vi "Periodic Tasks.vi"(8 "error in":errorcluster) -> ()   [LabVIEW 2012]
doc: "This VI runs in parallel to other tasks. It can contain as many user-defined periodic loops as you need. These can carry out PID or other sorts of timed response."
uses:
  <vilib>/Rock Robotics/SystemInterfaces/Utilities/FPGA_UtilitiesLED Source.ctl
  <vilib>/Rock Robotics/SystemInterfaces/Utilities/FPGA_UtilitiesLED State.ctl
  <vilib>/Rock Robotics/WPI/Solenoid/WPI_SolenoidValue.ctl
  Robot Global Data.vi
  <vilib>/Rock Robotics/WPI/Solenoid/WPI_SolenoidSetEnum.vi
  <vilib>/Rock Robotics/WPI/Compressor/WPI_CompressorGetSetRefNum.vi
panel:
  out "Angle":dbl
  out "Ave Voltage":dbl
  out "Voltage":dbl
  out "PickupErrort":errorcluster
  # "AnglePot"
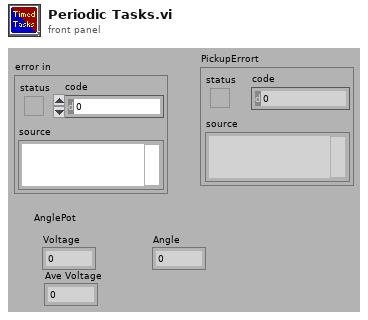
[diagram p1: front panel]
types:
  T1 = enum16{"Reset", "Ready", "Down", "Capture", "Lift", "Swing", "Release"}
  T2 = typedef "WPI_MotorControlDeviceRef.ctl" = cluster{"DeviceStatus":errorcluster, "Type":enum16{"PWM", "CAN"}, "PWM":cluster{"Digital Module":T3, "PWM Channel":T4, "DeadBand":T5}, "CAN":cluster{"Device Number":u8, "Control Mode":T6, "Semaphore":T7, "Max Vout":dbl}, "Invert":bool, "TransformRef":T8, "InvTransformRef":T8}
  T3 = typedef "FPGA_TypedefDigitalModule.ctl" = enum16{"Digital Module 1", "Digital Module 2"}
  T4 = typedef "FPGA_DIOPWMChannel.ctl" = enum8{"PWM 1", "PWM 2", "PWM 3", "PWM 4", "PWM 5", "PWM 6", "PWM 7", "PWM 8", "PWM 9", "PWM 10", "Invalid"}
  T5 = typedef "WPI_PWMDeadband.ctl" = cluster{"Name":string, "maxPositivePwm":i32, "minPositivePwm":i32, "centerPwm":i32, "maxNegativePwm":i32, "minNegativePwm":i32, "angularRange":u16}
  T6 = typedef "WPI_CANJaguar_ControlMode.ctl" = enum8{"Percent VBus", "Current", "Speed", "Position", "Voltage"}
  T7 = typedef "Semaphore RefNum" = refnum<k1>
  T8 = typedef "WPI_PWMTransform_ConPane.ctl" = refnum<vi>
  T9 = typedef "WPI_SolenoidDevRef.ctl" = cluster{"DevStatus":errorcluster, "Solenoid Module":T10, "Forward Solenoid Channel":T11, "Reverse Solenoid Channel":T11}
  T10 = typedef "FPGA_TypedefSolenoidModule.ctl" = enum16{"Solenoid Module 1", "Solenoid Module 2"}
  T11 = typedef "WPI_SolenoidChannel.ctl" = enum8{"Solenoid 1", "Solenoid 2", "Solenoid 3", "Solenoid 4", "Solenoid 5", "Solenoid 6", "Solenoid 7", "Solenoid 8", "Invalid"}
  T12 = typedef "WPI_AnalogChannelDevRef.ctl" = cluster{"DevStatus":errorcluster, "Analog Module":T13, "Analog Channel":T14}
  T13 = typedef "FPGA_TypedefAnalogModule.ctl" = enum16{"Analog Module 1", "Analog Module 2"}
  T14 = typedef "FPGA_AIChannel.ctl" = enum8{"AI 1", "AI 2", "AI 3", "AI 4", "AI 5", "AI 6", "AI 7", "AI 8", "Invalid"}
  T15 = typedef "FPGA_UtilitiesLED State.ctl" = enum16{"Off", "On", "Toggle"}
  T16 = typedef "FPGA_UtilitiesLED Source.ctl" = enum16{"User LED", "FPGA LED"}
  T17 = typedef "WPI_SolenoidValue.ctl" = enum16{"Off", "On", "Forward", "Reverse"}
  T18 = cluster{"Shoot":bool, "Enable_Targeting":bool, "Shooter":dbl, "LeadScrew":dbl, "Feed":bool, "SuctionCup":bool, "SuctionRotate":bool, "SuctionExtend":bool, "Pickup":bool, "PizzaBottom":bool, "PizzaMid":bool, "Pizza_top":bool}
  T19 = cluster{"Prox1":bool, "Prox2":bool, "Prox3":bool, "Frisbee_Catch":bool, "Frisbee_Side_Check":bool, "Shooter_Ready":bool, "LeadScrewEnd":bool}
  T20 = cluster{"PizzaLow":dbl, "PizzaMid":dbl, "PizzaTop":dbl}
  T21 = typedef "WPI_CompressorDevRef.ctl" = cluster{"DevStatus":errorcluster, "DigitalInputDevRef":T22, "RelayDevRef":T24}
  T22 = typedef "WPI_DigitalInputDevRef.ctl" = cluster{"DevStatus":errorcluster, "DIO Channel":T23, "Digital Module":T3}
  T23 = typedef "FPGA_DIOChannel.ctl" = enum8{"DIO 1", "DIO 2", "DIO 3", "DIO 4", "DIO 5", "DIO 6", "DIO 7", "DIO 8", "DIO 9", "DIO 10", "DIO 11", "DIO 12", "DIO 13", "DIO 14", "Invalid"}
  T24 = typedef "WPI_RelayDevRef.ctl" = cluster{"DevStatus":errorcluster, "Relay Channel":T25, "Digital Module":T3, "Relay Direction":T26}
  T25 = typedef "FPGA_DIORelayChannel.ctl" = enum8{"Relay 1", "Relay 2", "Relay 3", "Relay 4", "Relay 5", "Relay 6", "Relay 7", "Relay 8", "Invalid"}
  T26 = typedef "WPI_RelayDirection.ctl" = enum16{"Both directions", "Forward only", "Reverse only"}
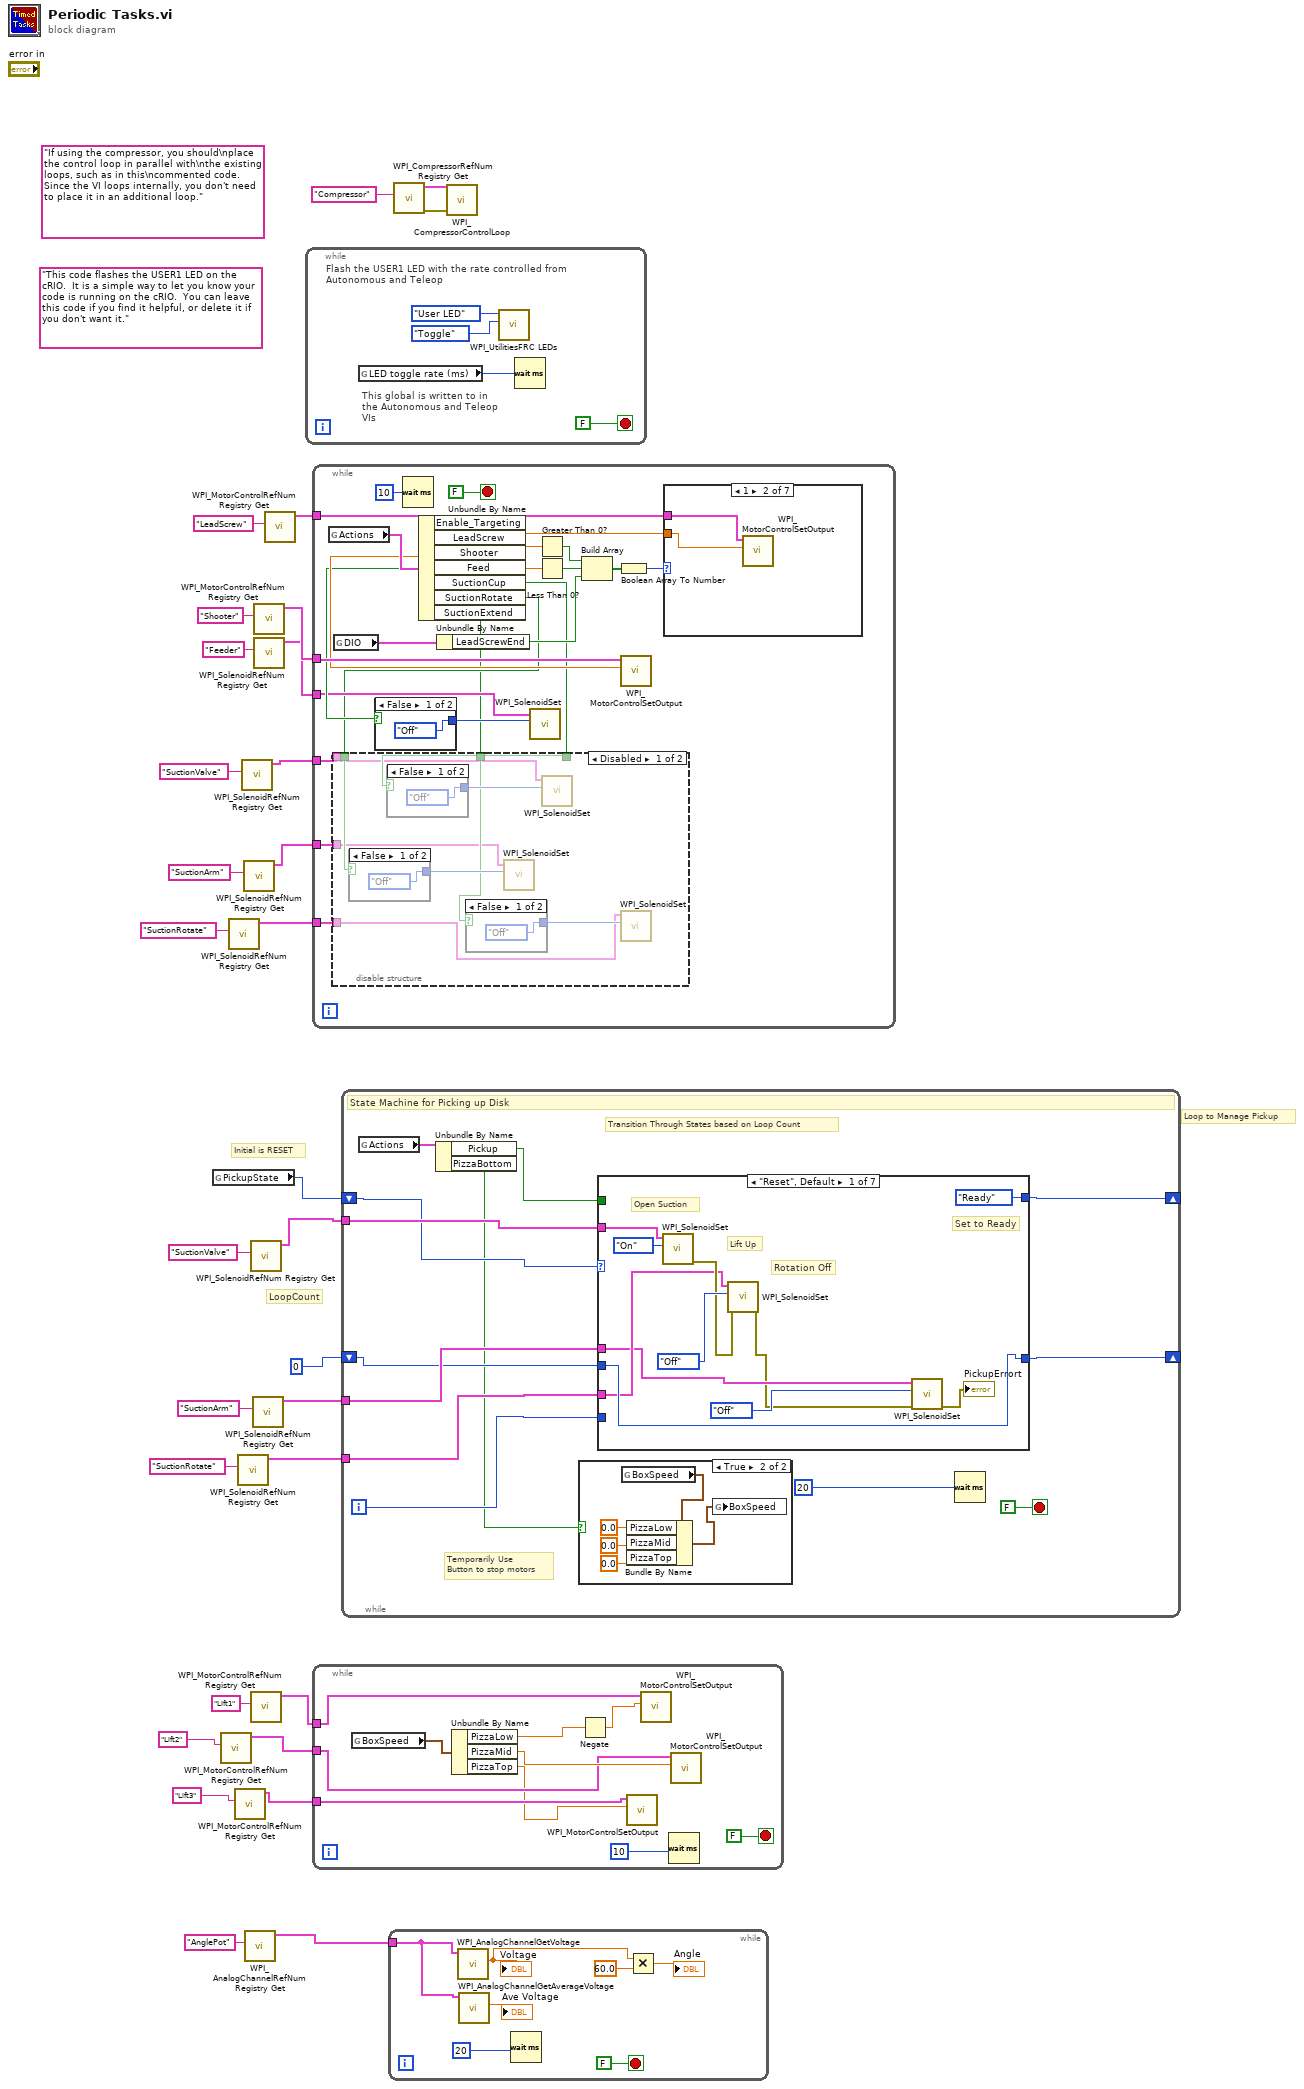
[diagram p0: block diagram]
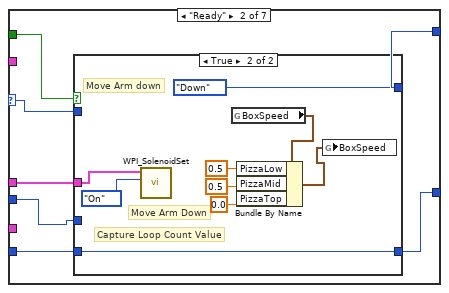
[diagram p3: hidden frame]
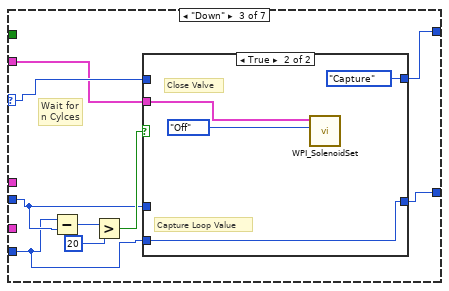
[diagram p5: hidden frame]
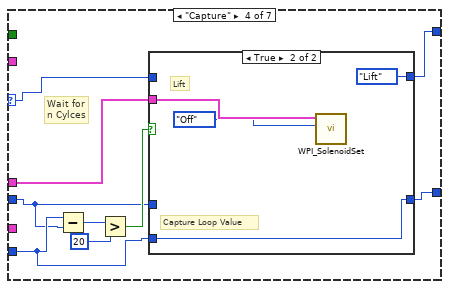
[diagram p7: hidden frame]
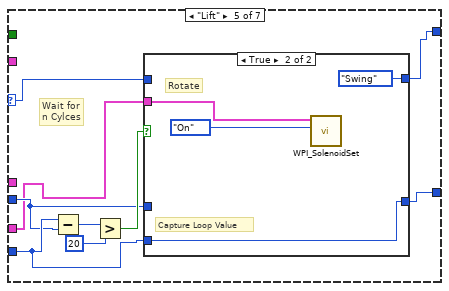
[diagram p9: hidden frame]
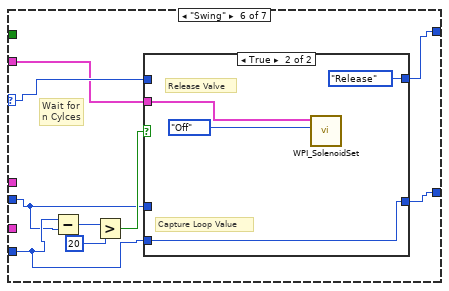
[diagram p11: hidden frame]
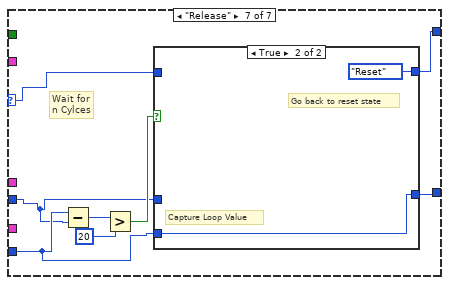
[diagram p13: hidden frame]
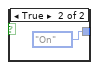
[diagram p15: hidden frame]
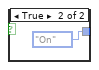
[diagram p16: hidden frame]
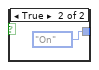
[diagram p17: hidden frame]
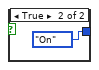
[diagram p19: hidden frame]
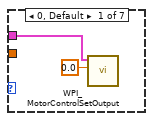
[diagram p20: hidden frame]
diagram:
  (unwired) "If using the compressor, you should\nplace the control loop in parallel with\nthe existing loops, such as in this\ncommented code. Since the VI loops internally, you don't need to place it in an additional loop."
  (unwired) "This code flashes the USER1 LED on the cRIO.  It is a simple way to let you know your code is running on the cRIO.  You can leave this code if you find it helpful, or delete it if you don't want it."
  # "LoopCount"
  # "Initial is RESET"
  # "Loop to Manage Pickup"
  n1 = global read "Robot Global Data.vi" "PickupState"() -> (w10:T1)
  n2 = call <vilib>:"WPI_MotorControlRefNum Registry Get.vi"("refnum name"="Lift2") -> ("MotorControlDevRef"=w5:T2)  [unwired: 9 in, 1 out]
  n3 = call <vilib>:"WPI_SolenoidRefNum Registry Get.vi"("refnum name"="SuctionRotate") -> ("SolenoidDevRef"=w17:T9)  [unwired: 9 in, 1 out]
  n4 = call <vilib>:"WPI_MotorControlRefNum Registry Get.vi"("refnum name"="Lift3") -> ("MotorControlDevRef"=w4:T2)  [unwired: 9 in, 1 out]
  n5 = call <vilib>:"WPI_SolenoidRefNum Registry Get.vi"("refnum name"="SuctionRotate") -> ("SolenoidDevRef"=w11:T9)  [unwired: 9 in, 1 out]
  n6 = call <vilib>:"WPI_SolenoidRefNum Registry Get.vi"("refnum name"="SuctionValve") -> ("SolenoidDevRef"=w19:T9)  [unwired: 9 in, 1 out]
  n7 = call <vilib>:"WPI_SolenoidRefNum Registry Get.vi"("refnum name"="SuctionArm") -> ("SolenoidDevRef"=w18:T9)  [unwired: 9 in, 1 out]
  n8 = call <vilib>:"WPI_AnalogChannelRefNum Registry Get.vi"("refnum name"="AnglePot") -> ("AIDeviceRef"=w1:T12)  [unwired: 9 in, 1 out]
  n9 = call <vilib>:"WPI_SolenoidRefNum Registry Get.vi"("refnum name"="SuctionValve") -> ("SolenoidDevRef"=w13:T9)  [unwired: 9 in, 1 out]
  n10 = call <vilib>:"WPI_MotorControlRefNum Registry Get.vi"("refnum name"="Lift1") -> ("MotorControlDevRef"=w6:T2)  [unwired: 9 in, 1 out]
  n11 = call <vilib>:"WPI_SolenoidRefNum Registry Get.vi"("refnum name"="SuctionArm") -> ("SolenoidDevRef"=w12:T9)  [unwired: 9 in, 1 out]
  n12 = call <vilib>:"WPI_MotorControlRefNum Registry Get.vi"("refnum name"="Shooter") -> ("MotorControlDevRef"=w25:T2)  [unwired: 9 in, 1 out]
  n13 = call <vilib>:"WPI_SolenoidRefNum Registry Get.vi"("refnum name"="Feeder") -> ("SolenoidDevRef"=w24:T9)  [unwired: 9 in, 1 out]
  n14 = call <vilib>:"WPI_MotorControlRefNum Registry Get.vi"("refnum name"="LeadScrew") -> ("MotorControlDevRef"=w27:T2)  [unwired: 9 in, 1 out]
  n15 = while {
    stop <- FALSE stop-if-true
    # "This global is written to in the Autonomous and Teleop VIs"
    # "Flash the USER1 LED with the rate controlled from Autonomous and Teleop"
    n16 = global read "Robot Global Data.vi" "LED toggle rate (ms)"() -> (w32:u32)
    n17 = call <vilib>:"WPI_UtilitiesFRC LEDs.vi"("State"=FPGA_UtilitiesLED_State."Toggle", "LED Type"=FPGA_UtilitiesLED_Source."User LED") -> ()  [unwired: 1 in, 9 out]
    n18 = Wait (ms)(milliseconds to wait=w32) -> ()  [unwired: 1 out]
  }
  n19 = while {
    tunnel: w27 -> [w49]
    tunnel: w25 -> [w48]
    tunnel: w24 -> [w42]
    tunnel: w19 -> [w38]
    tunnel: w18 -> [w37]
    tunnel: w17 -> [w36]
    stop <- FALSE stop-if-true
    n20 = global read "Robot Global Data.vi" "Actions"() -> (w47:T18)
    n21 = global read "Robot Global Data.vi" "DIO"() -> (w46:T19)
    n22 = Wait (ms)(milliseconds to wait=u32 10) -> ()  [unwired: 1 out]
    n23 = Unbundle By Name(w47) -> ("LeadScrew"=w51:dbl, "Shooter"=w45:dbl, "Feed"=w44:bool, "SuctionCup"=w41:bool, "SuctionRotate"=w40:bool, "SuctionExtend"=w39:bool)  [unwired: 1 out]
    n24 = disable-structure shown="Disabled" {
      disable-tunnel: w41 -> [w63 _]
      disable-tunnel: w40 -> [w62 _]
      disable-tunnel: w39 -> [w61 _]
      disable-tunnel: w38 -> [w60 _]
      disable-tunnel: w37 -> [w59 _]
      disable-tunnel: w36 -> [w58 _]
      frame Disabled {
        n25 = case shown="False" w62 {
          tunnel: [WPI_SolenoidValue."Off" ("Value") WPI_SolenoidValue."On" ("Value")] -> w65
          frame False {
          }
          frame True {
          }
        }
        n26 = case shown="False" w63 {
          tunnel: [WPI_SolenoidValue."Off" ("Value") WPI_SolenoidValue."On" ("Value")] -> w66
          frame False {
          }
          frame True {
          }
        }
        n27 = case shown="False" w61 {
          tunnel: [WPI_SolenoidValue."Off" ("Value") WPI_SolenoidValue."On" ("Value")] -> w64
          frame False {
          }
          frame True {
          }
        }
        n28 = call-poly <vilib>:"WPI_SolenoidSet.vi"("Value"=w65, "SolenoidDevRef"=w59) -> ()  [unwired: 8 in, 2 out]
        n29 = call-poly <vilib>:"WPI_SolenoidSet.vi"("Value"=w66, "SolenoidDevRef"=w60) -> ()  [unwired: 8 in, 2 out]
        n30 = call-poly <vilib>:"WPI_SolenoidSet.vi"("Value"=w64, "SolenoidDevRef"=w58) -> ()  [unwired: 8 in, 2 out]
      }
      frame Enabled {
      }
    }
    n31 = case shown="False" w44 {
      tunnel: [WPI_SolenoidValue."Off" ("Value") WPI_SolenoidValue."On" ("Value")] -> w43
      frame False {
      }
      frame True {
      }
    }
    n32 = Unbundle By Name(w46) -> ("LeadScrewEnd"=w50:bool)
    n33 = call-poly <vilib>:"WPI_SolenoidSet.vi"("Value"=w43, "SolenoidDevRef"=w42) -> ()  [unwired: 8 in, 2 out]
    n34 = Greater Than 0?(x=w51) -> (x > 0?=w54:bool)
    n35 = Less Than 0?(x=w51) -> (x < 0?=w55:bool)
    n36 = Build Array(w54, w55, w50) -> (w53:bool[])
    n37 = Boolean Array To Number(Boolean array=w53) -> (number=w52:u32)
    n38 = call <vilib>:"WPI_MotorControlSetOutput.vi"("Output"=w45, "MotorControlDevRef"=w48) -> ()  [unwired: 7 in, 3 out]
    n39 = case shown="1" w52 {
      tunnel: w51 -> [_ w78 w80 _ _ _ w87]
      tunnel: w49 -> [w75 w77 w79 w82 w84 w86 w88]
      frame 0, Default {
        n40 = call <vilib>:"WPI_MotorControlSetOutput.vi"("Output"=0.0, "MotorControlDevRef"=w75) -> ()  [unwired: 7 in, 3 out]
      }
      frame 1 {
        n41 = call <vilib>:"WPI_MotorControlSetOutput.vi"("Output"=w78, "MotorControlDevRef"=w77) -> ()  [unwired: 7 in, 3 out]
      }
      frame 2 {
        n42 = call <vilib>:"WPI_MotorControlSetOutput.vi"("Output"=w80, "MotorControlDevRef"=w79) -> ()  [unwired: 7 in, 3 out]
      }
      frame 3 {
        n43 = call <vilib>:"WPI_MotorControlSetOutput.vi"("Output"=0.0, "MotorControlDevRef"=w82) -> ()  [unwired: 7 in, 3 out]
      }
      frame 4 {
        n44 = call <vilib>:"WPI_MotorControlSetOutput.vi"("Output"=0.0, "MotorControlDevRef"=w84) -> ()  [unwired: 7 in, 3 out]
      }
      frame 5 {
        n45 = call <vilib>:"WPI_MotorControlSetOutput.vi"("Output"=0.0, "MotorControlDevRef"=w86) -> ()  [unwired: 7 in, 3 out]
      }
      frame 6 {
        n46 = call <vilib>:"WPI_MotorControlSetOutput.vi"("Output"=w87, "MotorControlDevRef"=w88) -> ()  [unwired: 7 in, 3 out]
      }
    }
  }
  n47 = while {
    tunnel: w6 -> [w95]
    tunnel: w5 -> [w94]
    tunnel: w4 -> [w93]
    stop <- FALSE stop-if-true
    n48 = global read "Robot Global Data.vi" "BoxSpeed"() -> (w97:T20)
    n49 = Unbundle By Name(w97) -> ("PizzaLow"=w90:dbl, "PizzaMid"=w96:dbl, "PizzaTop"=w92:dbl)
    n50 = Negate(x=w90) -> (-x=w89:dbl)
    n51 = call <vilib>:"WPI_MotorControlSetOutput.vi"("Output"=w92, "MotorControlDevRef"=w93) -> ()  [unwired: 7 in, 3 out]
    n52 = call <vilib>:"WPI_MotorControlSetOutput.vi"("Output"=w89, "MotorControlDevRef"=w95) -> ()  [unwired: 7 in, 3 out]
    n53 = Wait (ms)(milliseconds to wait=u32 10) -> ()  [unwired: 1 out]
    n54 = call <vilib>:"WPI_MotorControlSetOutput.vi"("Output"=w96, "MotorControlDevRef"=w94) -> ()  [unwired: 7 in, 3 out]
  }
  n55 = while {
    tunnel: w13 -> [w109]
    tunnel: w12 -> [w108]
    tunnel: w11 -> [w107]
    shift-right: [w106] -> _
    shift-left: w10 -> [w105]
    shift-right: [w100] -> _
    shift-left: 0 -> [w101]
    i -> [w102]
    stop <- FALSE stop-if-true
    # "Temporarily Use\nButton to stop motors"
    # "Transition Through States based on Loop Count"
    # "State Machine for Picking up Disk"
    n56 = global read "Robot Global Data.vi" "Actions"() -> (w104:T18)
    n57 = Unbundle By Name(w104) -> ("Pickup"=w103:bool, "PizzaBottom"=w99:bool)
    n58 = case shown="True" w99 {
      frame False {
      }
      frame True {
        n59 = global read "Robot Global Data.vi" "BoxSpeed"() -> (w112:T20)
        n60 = Bundle By Name(cluster=w112, "PizzaLow"=0.0, "PizzaMid"=0.0, "PizzaTop"=0.0) -> (w116:T20)
        n61 = global write "Robot Global Data.vi" "BoxSpeed"(w116) -> ()
      }
    }
    n62 = case shown="\"Reset\", Default" w105 {
      selector: w105 -> [_ w128 w149 w166 w177 w192 w208]
      tunnel: w109 -> [w127 _ w146 _ _ w191 _]
      tunnel: w108 -> [w118 w132 _ w163 _ _ _]
      tunnel: w107 -> [w119 _ _ _ w176 _ _]
      tunnel: [T1."Ready" ("PickupState") w133 w148 w162 w178 w196 w207] -> w106
      tunnel: w103 -> [_ w134 _ _ _ _ _]
      tunnel: w102 -> [_ w131 w147 w165 w181 w194 w210]
      tunnel: w101 -> [w120 w129 w151 w164 w180 w193 w209]
      tunnel: [w120 w130 w150 w161 w179 w195 w206] -> w100
      frame "Reset", Default {
        # "Set to Ready"
        # "Rotation Off"
        # "Lift Up"
        # "Open Suction"
        n63 = call-poly <vilib>:"WPI_SolenoidSet.vi"("Value"=WPI_SolenoidValue."On", "SolenoidDevRef"=w127) -> ("error out"=w124:errorcluster)  [unwired: 8 in, 1 out]
        n64 = call-poly <vilib>:"WPI_SolenoidSet.vi"("error in (no error)"=w124, "Value"=WPI_SolenoidValue."Off", "SolenoidDevRef"=w119) -> ("error out"=w117:errorcluster)  [unwired: 7 in, 1 out]
        n65 = call-poly <vilib>:"WPI_SolenoidSet.vi"("error in (no error)"=w117, "Value"=WPI_SolenoidValue."Off", "SolenoidDevRef"=w118) -> ("error out"=→"PickupErrort":errorcluster)  [unwired: 7 in, 1 out]
      }
      frame "Ready" {
        n66 = case shown="True" w134 {
          tunnel: [w135 T1."Down" ("PickupState")] -> w133
          tunnel: w132 -> [_ w144]
          tunnel: w131 -> [_ w142]
          tunnel: [w136 w142] -> w130
          tunnel: w129 -> [w136 _]
          tunnel: w128 -> [w135 _]
          frame False {
            # "Pass state\nand Loop\nCount"
          }
          frame True {
            # "Move Arm down"
            # "Capture Loop Count Value"
            # "Move Arm Down"
            n67 = call-poly <vilib>:"WPI_SolenoidSet.vi"("Value"=WPI_SolenoidValue."On", "SolenoidDevRef"=w144) -> ()  [unwired: 8 in, 2 out]
            n68 = global read "Robot Global Data.vi" "BoxSpeed"() -> (w141:T20)
            n69 = Bundle By Name(cluster=w141, "PizzaLow"=0.5, "PizzaMid"=0.5, "PizzaTop"=0.0) -> (w137:T20)
            n70 = global write "Robot Global Data.vi" "BoxSpeed"(w137) -> ()
          }
        }
      }
      frame "Down" {
        # "Wait for\nn Cylces"
        n71 = Subtract(x=w147, y=w151) -> (x-y=w154:i32)
        n72 = Greater?(x=w154, y=20) -> (0:w152:bool)
        n73 = case shown="True" w152 {
          tunnel: w151 -> [w156 _]
          tunnel: [w156 w160] -> w150
          tunnel: w149 -> [w155 _]
          tunnel: [w155 T1."Capture" ("PickupState")] -> w148
          tunnel: w147 -> [_ w160]
          tunnel: w146 -> [_ w159]
          frame False {
            # "Keep Waiting"
          }
          frame True {
            # "Capture Loop Value"
            # "Close Valve"
            n74 = call-poly <vilib>:"WPI_SolenoidSet.vi"("Value"=WPI_SolenoidValue."Off", "SolenoidDevRef"=w159) -> ()  [unwired: 8 in, 2 out]
          }
        }
      }
      frame "Capture" {
        # "Wait for\nn Cylces"
        n75 = Subtract(x=w165, y=w164) -> (x-y=w169:i32)
        n76 = Greater?(x=w169, y=20) -> (0:w167:bool)
        n77 = case shown="True" w167 {
          tunnel: w164 -> [w171 _]
          tunnel: [w171 w175] -> w161
          tunnel: w166 -> [w170 _]
          tunnel: [w170 T1."Lift" ("PickupState")] -> w162
          tunnel: w165 -> [_ w175]
          tunnel: w163 -> [_ w174]
          frame False {
            # "Keep Waiting"
          }
          frame True {
            # "Capture Loop Value"
            # "Lift"
            n78 = call-poly <vilib>:"WPI_SolenoidSet.vi"("Value"=WPI_SolenoidValue."Off", "SolenoidDevRef"=w174) -> ()  [unwired: 8 in, 2 out]
          }
        }
      }
      frame "Lift" {
        # "Wait for\nn Cylces"
        n79 = Subtract(x=w181, y=w180) -> (x-y=w184:i32)
        n80 = Greater?(x=w184, y=20) -> (0:w182:bool)
        n81 = case shown="True" w182 {
          tunnel: w180 -> [w186 _]
          tunnel: [w186 w190] -> w179
          tunnel: w177 -> [w185 _]
          tunnel: [w185 T1."Swing" ("PickupState")] -> w178
          tunnel: w181 -> [_ w190]
          tunnel: w176 -> [_ w189]
          frame False {
            # "Keep Waiting"
          }
          frame True {
            # "Capture Loop Value"
            # "Rotate"
            n82 = call-poly <vilib>:"WPI_SolenoidSet.vi"("Value"=WPI_SolenoidValue."On", "SolenoidDevRef"=w189) -> ()  [unwired: 8 in, 2 out]
          }
        }
      }
      frame "Swing" {
        # "Wait for\nn Cylces"
        n83 = Subtract(x=w194, y=w193) -> (x-y=w199:i32)
        n84 = Greater?(x=w199, y=20) -> (0:w197:bool)
        n85 = case shown="True" w197 {
          tunnel: w193 -> [w201 _]
          tunnel: [w201 w205] -> w195
          tunnel: w192 -> [w200 _]
          tunnel: [w200 T1."Release" ("PickupState")] -> w196
          tunnel: w194 -> [_ w205]
          tunnel: w191 -> [_ w204]
          frame False {
            # "Keep Waiting"
          }
          frame True {
            # "Capture Loop Value"
            # "Release Valve"
            n86 = call-poly <vilib>:"WPI_SolenoidSet.vi"("Value"=WPI_SolenoidValue."Off", "SolenoidDevRef"=w204) -> ()  [unwired: 8 in, 2 out]
          }
        }
      }
      frame "Release" {
        # "Wait for\nn Cylces"
        n87 = Subtract(x=w210, y=w209) -> (x-y=w213:i32)
        n88 = Greater?(x=w213, y=20) -> (0:w211:bool)
        n89 = case shown="True" w211 {
          tunnel: w209 -> [w215 _]
          tunnel: [w215 w217] -> w206
          tunnel: w208 -> [w214 _]
          tunnel: [w214 T1."Reset" ("PickupState")] -> w207
          tunnel: w210 -> [_ w217]
          frame False {
            # "Keep Waiting"
          }
          frame True {
            # "Go back to reset state"
            # "Capture Loop Value"
          }
        }
      }
    }
    n90 = Wait (ms)(milliseconds to wait=u32 20) -> ()  [unwired: 1 out]
  }
  n91 = while {
    tunnel: w1 -> [w224]
    stop <- FALSE stop-if-true
    n92 = call <vilib>:"WPI_AnalogChannelGetVoltage.vi"("AIDeviceRef"=w224) -> ("Voltage"=w220:dbl)  [unwired: 8 in, 2 out]
    "Voltage" <- w220
    n93 = call <vilib>:"WPI_AnalogChannelGetAverageVoltage.vi"("AIDeviceRef"=w224) -> ("Voltage"=→"Ave Voltage":dbl)  [unwired: 8 in, 2 out]
    n94 = Wait (ms)(milliseconds to wait=u32 20) -> ()  [unwired: 1 out]
    n95 = Multiply(x=w220, y=60.0) -> (x*y=→"Angle":dbl)
  }
  n96 = call <vilib>:"WPI_CompressorRefNum Registry Get.vi"("refnum name"="Compressor") -> ("error out"=w29:errorcluster, "CompressorDevRef"=w31:T21)  [unwired: 9 in]
  n97 = call <vilib>:"WPI_CompressorControlLoop.vi"("error in (no error)"=w29, "CompressorDevRef"=w31) -> ()  [unwired: 10 in]
